vi "Load Settings from XML.vi"(8 "error in (no error)":errorcluster, 11 "Settings in":T1={"Connection Configuration"={"Data source"=enum."Serial port", "Connection info"={"VISA resource name"="COM 1", "Baud rate"=9600, "data bits"=8, "stop bits"=0, "parity (0:none)"=enum."None", "flow control (0:none)"=0, "timeout (10sec)"=10000, "termination char\n(0xA = '\\n' = LF) "=10, "Enable Termination\nChar (T)"=TRUE}, "Protocol info"={"Temination char"=255, "Escape char"=254}, "Internet server"={"Web page telemetry"="", "Web page gps"=""}, "Data format"=enum."IDRA data"}, "Logging Configuration"={"Log File Base Path"=path "", "TDMS File Reference"=refnum, "Data format"=enum."IDRA data"}, "Maps config"={"Real-time map config"={"Config path"=path "", "Image path"=path ""}, "Mini map config"={"Config path"=path "", "Image path"=path ""}}, "Data format"=enum."IDRA data"} {"Connection Configuration"."Connection info"."flow control (0:none)" items=["None", "XON/XOFF", "RTS/CTS", "XON/XOFF & RTS/CTS", "DTR/DSR", "XON/XOFF & DTR/DSR"]}) -> (0 "error out":errorcluster, 3 "Settings out":T1={"Connection Configuration"={"Data source"=enum."Serial port", "Connection info"={"VISA resource name"="COM 1", "Baud rate"=9600, "data bits"=8, "stop bits"=0, "parity (0:none)"=enum."None", "flow control (0:none)"=0, "timeout (10sec)"=10000, "termination char\n(0xA = '\\n' = LF) "=10, "Enable Termination\nChar (T)"=TRUE}, "Protocol info"={"Temination char"=255, "Escape char"=254}, "Internet server"={"Web page telemetry"="", "Web page gps"=""}, "Data format"=enum."IDRA data"}, "Logging Configuration"={"Log File Base Path"=path "", "TDMS File Reference"=refnum, "Data format"=enum."IDRA data"}, "Maps config"={"Real-time map config"={"Config path"=path "", "Image path"=path ""}, "Mini map config"={"Config path"=path "", "Image path"=path ""}}, "Data format"=enum."IDRA data"} {"Connection Configuration"."Connection info"."flow control (0:none)" items=["None", "XON/XOFF", "RTS/CTS", "XON/XOFF & RTS/CTS", "DTR/DSR", "XON/XOFF & DTR/DSR"]})   [LabVIEW 2015, in "Settings.lvlib"]
doc: "Attempts to load previous user specified settings from an XML file.\n\nThis VI will not generate an error. If a suitable XML file can't be loaded and parsed then it will simply return the default settings."
uses:
  Settings.lvlib
  Settings.ctl
  Acquisition/Hardware Configuration.ctl
  Logging/Logging Configuration.ctl
  My Graphs/Gps Map Graph config.ctl
  <vilib>/Utility/xml.llb/Read From XML File(string).vi
  <vilib>/Utility/xml.llb/Write to XML File(string).vi
  Acquisition/Acquisition.lvlib
  Logging/Logging.lvlib
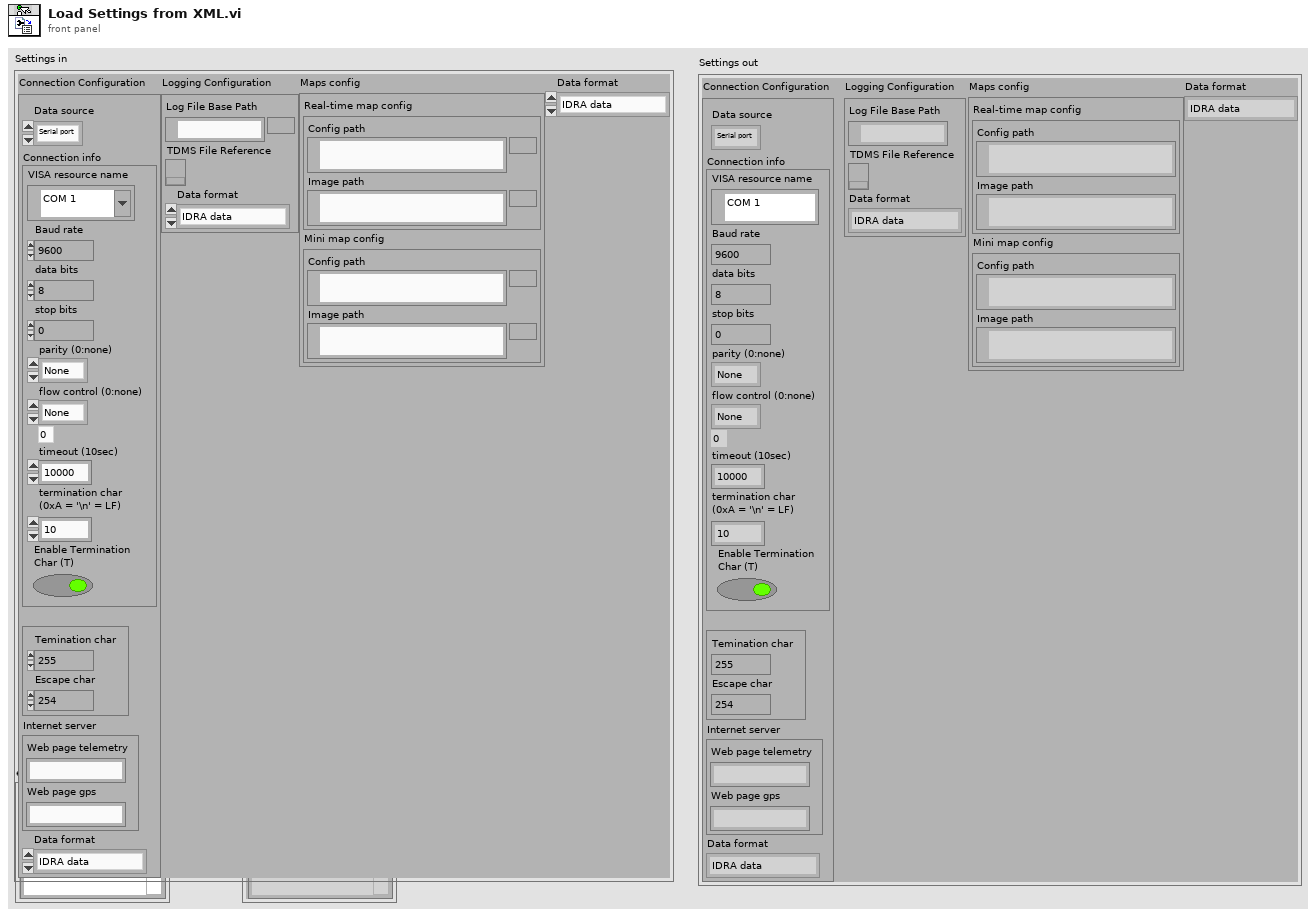
[diagram p1: front panel]
types:
  T1 = typedef "Settings.lvlib/Settings.ctl" = cluster{"Connection Configuration":T2, "Logging Configuration":T3, "Maps config":cluster{"Real-time map config":T4, "Mini map config":T4}, "Data format":enum16{"IDRA data", "XAM data"}}
  T2 = typedef "Acquisition.lvlib/Hardware Configuration.ctl" = cluster{"Data source":enum16{"Serial port", "Simulated data", "Web page JSON"}, "Connection info":cluster{"VISA resource name":refnum<visa-resource-name>, "Baud rate":u32, "data bits":u16, "stop bits":u16, "parity (0:none)":enum16{"None", "Odd", "Even", "Mark", "Space"}, "flow control (0:none)":u16, "timeout (10sec)":u32, "termination char\n(0xA = '\\n' = LF) ":u8, "Enable Termination\nChar (T)":bool}, "Protocol info":cluster{"Temination char":u8, "Escape char":u8}, "Internet server":cluster{"Web page telemetry":string, "Web page gps":string}, "Data format":enum16{"IDRA data", "XAM data"}}
  T3 = typedef "Logging.lvlib/Logging Configuration.ctl" = cluster{"Log File Base Path":path, "TDMS File Reference":refnum<k34>, "Data format":enum16{"IDRA data", "XAM data"}}
  T4 = typedef "Gps Map Graph config.ctl" = cluster{"Config path":path, "Image path":path}
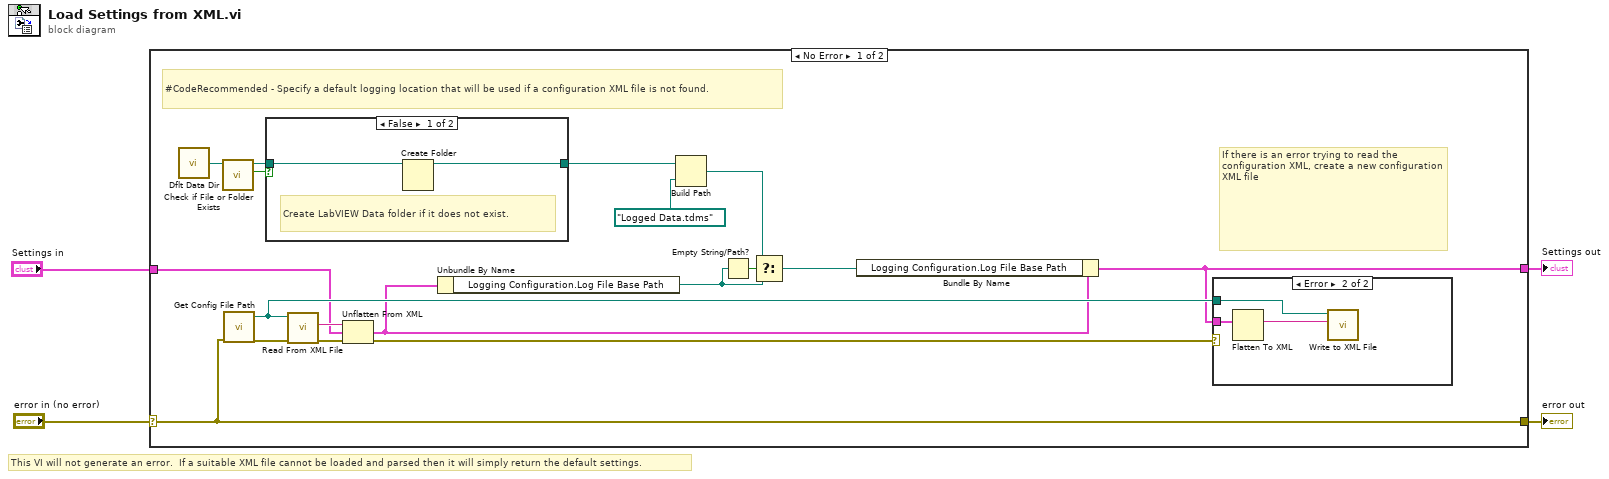
[diagram p0: block diagram]
diagram:
  # "This VI will not generate an error.  If a suitable XML file cannot be loaded and parsed then it will simply return the default settings."
  n1 = case shown="No Error" "error in (no error)" {
    selector: "error in (no error)" -> [w20 w30]
    tunnel: [w20 w30] -> w3
    tunnel: "Settings in" -> [w15 w29]
    tunnel: [w9 w29] -> w1
    frame No Error {
      # "If there is an error trying to read the configuration XML, create a new configuration XML file"
      # "#CodeRecommended - Specify a default logging location that will be used if a configuration XML file is not found."
      n2 = call <vilib>:"Dflt Data Dir.vi"() -> ("App:Default Data Directory"=w8:path)
      n3 = call <vilib>:"Check if File or Folder Exists.vi"("path"=w8) -> ("file or folder exists?"=w7:bool, "dup path"=w6:path)  [unwired: 8 in, 1 out]
      n4 = call "Get Config File Path.vi"("error in (no error)"=w20) -> ("error out"=w22:errorcluster, "XML File Path"=w18:path)  [unwired: 9 in]
      n5 = case shown="False" w7 {
        tunnel: w6 -> [w24 w25]
        tunnel: [w23 w25] -> w5
        frame False {
          # "Create LabVIEW Data folder if it does not exist."
          n6 = Create Folder(path (use dialog)=w24) -> (created path=w23:path)  [unwired: 2 in, 2 out]
        }
        frame True {
        }
      }
      n7 = call-poly <vilib>:"Read From XML File.vi"("error in (no error)"=w22, "XML File Path"=w18) -> ("error out"=w17:errorcluster, "XML Elements"=w21:string)  [unwired: 7 in, 1 out]
      n8 = Unflatten From XML(xml string=w21, type=w15, error in (no error)=w17) -> (value=w11:T1, error out=w16:errorcluster)
      n9 = Unbundle By Name(w11) -> ("Logging Configuration.Log File Base Path"=w13:path)
      n10 = Build Path(base path=w5, name or relative path=path "Logged Data.tdms" ("App:Default Data Directory")) -> (appended path=w12:path)
      n11 = Empty String/Path?(string/path=w13) -> (empty?=w14:bool)
      n12 = Select(t=w12, s=w14, f=w13) -> (s? t:f=w10:path)
      n13 = Bundle By Name(cluster=w11, "Logging Configuration.Log File Base Path"=w10) -> (w9:T1)
      n14 = case shown="Error" w16 {
        tunnel: w9 -> [_ w28]
        tunnel: w18 -> [_ w26]
        frame No Error {
        }
        frame Error {
          n15 = Flatten To XML(anything=w28) -> (xml string=w27:string)
          n16 = call-poly <vilib>:"Write to XML File.vi"("XML Input"=w27, "XML File Path"=w26) -> ()  [unwired: 7 in, 3 out]
        }
      }
    }
    frame Error {
    }
  }
  "error out" <- w3
  "Settings out" <- w1
